vi "MTM2_acceptCommand_start.vi"(8 "error in (no error)":errorcluster, 11 "command_start_Ctl":T1={"private_rcvStamp"=0.0, "settingsToApply"="                                                                                                                                                                                                                                                                "}) -> (0 "error out":errorcluster, 2 "function return":i32, 3 "command_start_Ctl out":T1={"private_rcvStamp"=0.0, "settingsToApply"="                                                                                                                                                                                                                                                                "})   [LabVIEW 2018, in "SALLV_MTM2.lvlib"]
doc: "int MTM2_shm_acceptCommand_startLV(MTM2_command_startLV *command_start_Ctl );"
uses:
  DataTypes/command_start.ctl
  SALLV_MTM2.lvlib
  SALLV_MTM2.so
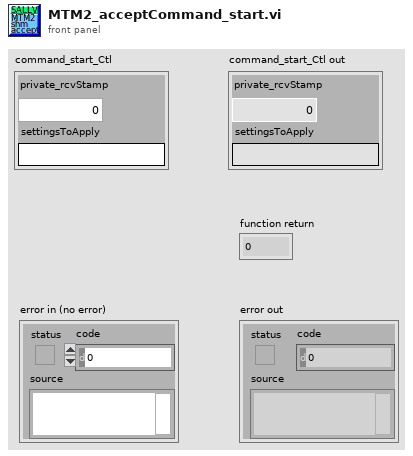
[diagram p1: front panel]
types:
  T1 = typedef "SALLV_MTM2.lvlib/command_start.ctl" = cluster{"private_rcvStamp":dbl, "settingsToApply":string}
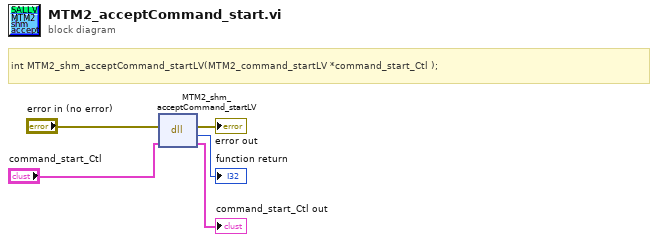
[diagram p0: block diagram]
diagram:
  # "int MTM2_shm_acceptCommand_startLV(MTM2_command_startLV *command_start_Ctl );"
  n1 = dll-call lib="home/ttsai/Documents/salTestLabViewApi/SALLV_MTM2/SALLV_MTM2.*" fn="MTM2_shm_acceptCommand_startLV"(error in="error in (no error)", "command_start_Ctl"="command_start_Ctl") -> (error out=→"error out":errorcluster, →"function return":i32, "command_start_Ctl"=→"command_start_Ctl out":T1)  [unwired: 2 in, 1 out]
